vi "calcCompensatorOutput.vi"(6 "reinitializeIsTrue":bool, 8 "error in (no error)":errorcluster, 9 "Force Measured":T2 min=-888.0 max=888.0 format="%.2f", 10 "Force Setpoint":T2 min=-888.0 max=888.0 format="%.2f", 11 "FlowControlValveCompensator in":refnum<class "FlowControlValveCompensator.lvclass">) -> (0 "error out":errorcluster, 2 "Flow Control Valve Setpoint":T1 min=-888.0 max=888.0 format="%.2f", 3 "FlowControlValveCompensator out":refnum<class "FlowControlValveCompensator.lvclass">)   [LabVIEW 2013, in "FlowControlValveCompensator.lvclass"]
uses:
  FlowControlValveCompensator.lvclass
  Typedefs/ForceSetpoint.ctl
  Typedefs/FlowControlValveSetpoint.ctl
  FlowControlValveCompensator.lvclass/FlowControlValveCompensator.ctl
  <vilib>/addons/control/pid/NI_PID_pid.lvlib
  Typedefs/FAMTTypedefs.lvlib
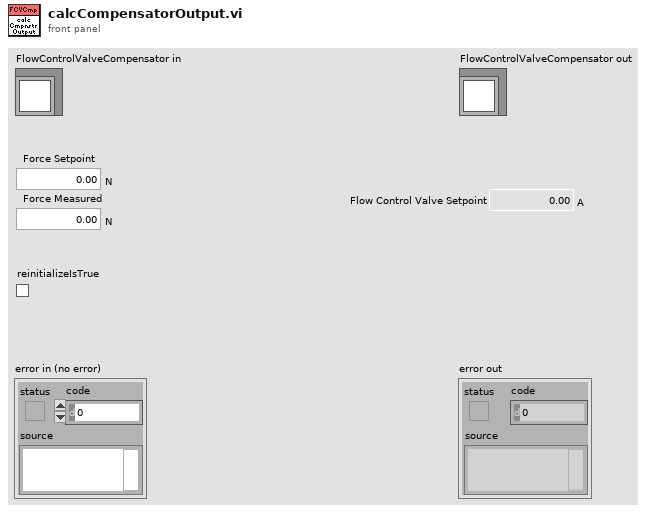
[diagram p1: front panel]
types:
  T1 = typedef "FAMTTypedefs.lvlib/FlowControlValveSetpoint.ctl" = dbl[unit]
  T2 = typedef "FAMTTypedefs.lvlib/ForceSetpoint.ctl" = dbl[unit]
  T3 = typedef "PIDGains.ctl" = cluster{"Proportional Gain (Kc)":dbl, "Integral Time (Ti, min)":dbl, "Derivative Time (Td, min)":dbl}
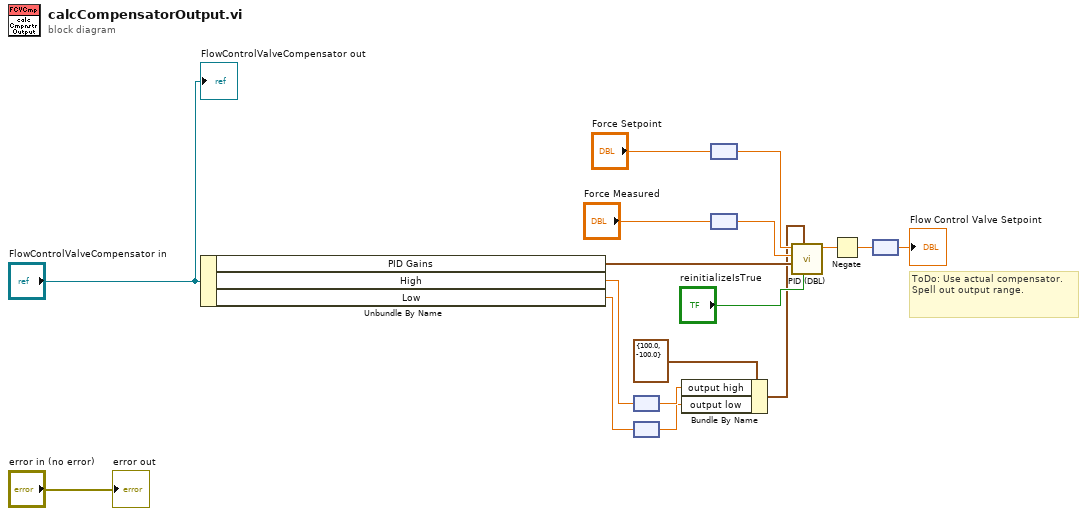
[diagram p0: block diagram]
diagram:
  # "ToDo: Use actual compensator.\nSpell out output range."
  n1 = Unbundle By Name("FlowControlValveCompensator in") -> ("PID Gains"=w11:T3, "High"=w4:dbl[unit], "Low"=w2:dbl[unit])
  n2 = node(w4) -> (w3:dbl)
  n3 = node(w2) -> (w1:dbl)
  n4 = Bundle By Name(cluster=cluster{"output high":dbl, "output low":dbl} {"output high"=100.0, "output low"=-100.0} ("output range"), "output high"=w3, "output low"=w1) -> (w5:cluster{"output high":dbl, "output low":dbl})
  n5 = node("Force Setpoint") -> (w15:dbl)
  n6 = node("Force Measured") -> (w16:dbl)
  n7 = call <vilib>:"PID (DBL).vi"("reinitialize? (F)"="reinitializeIsTrue", "output range"=w5, "PID gains"=w11, "process variable"=w16, "setpoint"=w15) -> ("output"=w12:dbl)  [unwired: 5 in, 1 out]
  n8 = Negate(x=w12) -> (-x=w13:dbl)
  n9 = node(w13) -> (→"Flow Control Valve Setpoint":dbl[unit])
  "error out" <- "error in (no error)"
  "FlowControlValveCompensator out" <- "FlowControlValveCompensator in"
